vi "Spatial Dual Decode Packet 29 (SubVI).vi"(11 "Packet 29 Bytes In":u8[](array[numeric])) -> (3 "Packet 29 Decoded":T1)   [LabVIEW 2019, in "SpatialDual_Parsers.lvlib"]
uses:
  SpatialDual_Parsers.lvlib
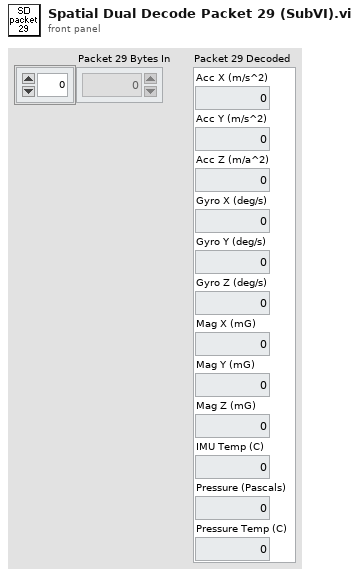
[diagram p1: front panel]
types:
  T1 = cluster{"Acc X (m/s^2)":sgl, "Acc Y (m/s^2)":sgl, "Acc Z (m/a^2)":sgl, "Gyro X (deg/s)":sgl, "Gyro Y (deg/s)":sgl, "Gyro Z (deg/s)":sgl, "Mag X (mG)":sgl, "Mag Y (mG)":sgl, "Mag Z (mG)":sgl, "IMU Temp (C)":sgl, "Pressure (Pascals)":sgl, "Pressure Temp (C)":sgl}
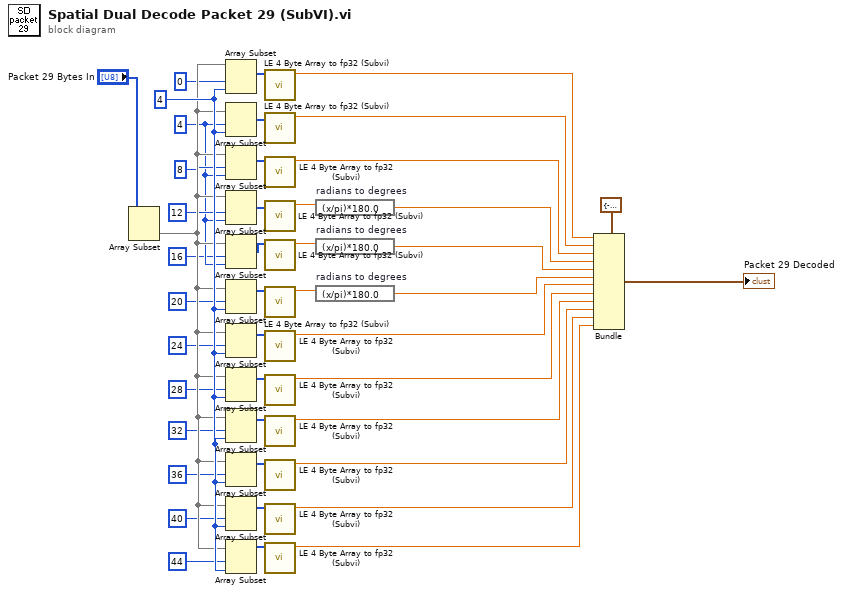
[diagram p0: block diagram]
diagram:
  w14 = 4 ("index")
  w22 = 4 ("index")
  n1 = Array Subset(array="Packet 29 Bytes In") -> (w21:u8[])  [unwired: 2 in]
  n2 = Array Subset(array=w21, index=0, length=w22) -> (w26:u8[])
  n3 = Array Subset(array=w21, index=w14, length=w22) -> (w23:u8[])
  n4 = Array Subset(array=w21, index=8, length=w14) -> (w27:u8[])
  n5 = Array Subset(array=w21, index=12, length=w14) -> (w24:u8[])
  n6 = Array Subset(array=w21, index=16, length=w14) -> (w25:u8[])
  n7 = Array Subset(array=w21, index=20, length=w22) -> (w11:u8[])
  n8 = Array Subset(array=w21, index=24, length=w22) -> (w8:u8[])
  n9 = Array Subset(array=w21, index=28, length=w22) -> (w7:u8[])
  n10 = Array Subset(array=w21, index=32, length=w22) -> (w5:u8[])
  n11 = Array Subset(array=w21, index=36, length=w22) -> (w2:u8[])
  n12 = Array Subset(array=w21, index=40, length=w22) -> (w1:u8[])
  n13 = Array Subset(array=w21, index=44, length=w22) -> (w19:u8[])
  n14 = call "LE 4 Byte Array to fp32 (Subvi).vi"("4 Bytes in"=w26) -> ("fp32 Out"=w32:sgl)  [unwired: 8 in]
  n15 = call "LE 4 Byte Array to fp32 (Subvi).vi"("4 Bytes in"=w23) -> ("fp32 Out"=w33:sgl)  [unwired: 8 in]
  n16 = call "LE 4 Byte Array to fp32 (Subvi).vi"("4 Bytes in"=w27) -> ("fp32 Out"=w34:sgl)  [unwired: 8 in]
  n17 = call "LE 4 Byte Array to fp32 (Subvi).vi"("4 Bytes in"=w24) -> ("fp32 Out"=w28:sgl)  [unwired: 8 in]
  n18 = call "LE 4 Byte Array to fp32 (Subvi).vi"("4 Bytes in"=w25) -> ("fp32 Out"=w29:sgl)  [unwired: 8 in]
  n19 = call "LE 4 Byte Array to fp32 (Subvi).vi"("4 Bytes in"=w11) -> ("fp32 Out"=w30:sgl)  [unwired: 8 in]
  n20 = call "LE 4 Byte Array to fp32 (Subvi).vi"("4 Bytes in"=w8) -> ("fp32 Out"=w38:sgl)  [unwired: 8 in]
  n21 = call "LE 4 Byte Array to fp32 (Subvi).vi"("4 Bytes in"=w7) -> ("fp32 Out"=w39:sgl)  [unwired: 8 in]
  n22 = call "LE 4 Byte Array to fp32 (Subvi).vi"("4 Bytes in"=w5) -> ("fp32 Out"=w40:sgl)  [unwired: 8 in]
  n23 = call "LE 4 Byte Array to fp32 (Subvi).vi"("4 Bytes in"=w2) -> ("fp32 Out"=w41:sgl)  [unwired: 8 in]
  n24 = call "LE 4 Byte Array to fp32 (Subvi).vi"("4 Bytes in"=w1) -> ("fp32 Out"=w42:sgl)  [unwired: 8 in]
  n25 = call "LE 4 Byte Array to fp32 (Subvi).vi"("4 Bytes in"=w19) -> ("fp32 Out"=w43:sgl)  [unwired: 8 in]
  n26 = expression code="(x/pi)*180.0" "radians to degrees"(w28) -> (w35:sgl)
  n27 = expression code="(x/pi)*180.0" "radians to degrees"(w29) -> (w36:sgl)
  n28 = expression code="(x/pi)*180.0" "radians to degrees"(w30) -> (w37:sgl)
  n29 = Bundle(cluster=T1 {"Acc X (m/s^2)"=-0.109794155, "Acc Y (m/s^2)"=-0.8886328, "Acc Z (m/a^2)"=-9.684429, "Gyro X (deg/s)"=2.2360516, "Gyro Y (deg/s)"=0.09974347, "Gyro Z (deg/s)"=-0.21773216, "Mag X (mG)"=83.319534, "Mag Y (mG)"=125.152664, "Mag Z (mG)"=404.77298, "IMU Temp (C)"=44.660156, "Pressure (Pascals)"=101860.055, "Pressure Temp (C)"=44.46} ("Cluster"), "Acc X (m/s^2)"=w32, "Acc Y (m/s^2)"=w33, "Acc Z (m/a^2)"=w34, "Gyro X (deg/s)"=w35, "Gyro Y (deg/s)"=w36, "Gyro Z (deg/s)"=w37, "Mag X (mG)"=w38, "Mag Y (mG)"=w39, "Mag Z (mG)"=w40, "IMU Temp (C)"=w41, "Pressure (Pascals)"=w42, "Pressure Temp (C)"=w43) -> (→"Packet 29 Decoded":T1)
